vi "Read IMAQ Session.vi"(8 "error in (no error)":errorcluster, 10 "Camera Name":string, 11 "Gantry Class in":refnum<class "Gantry.lvclass">) -> (0 "error out":errorcluster, 2 "IMAQ Session":T1, 3 "Gantry Class out":refnum<class "Gantry.lvclass">)   [LabVIEW 2017, in "Gantry.lvclass"]
uses:
  Gantry.lvclass
  <vilib>/userdefined/High Color/IMAQdx.ctl
  Gantry.lvclass/Gantry.ctl
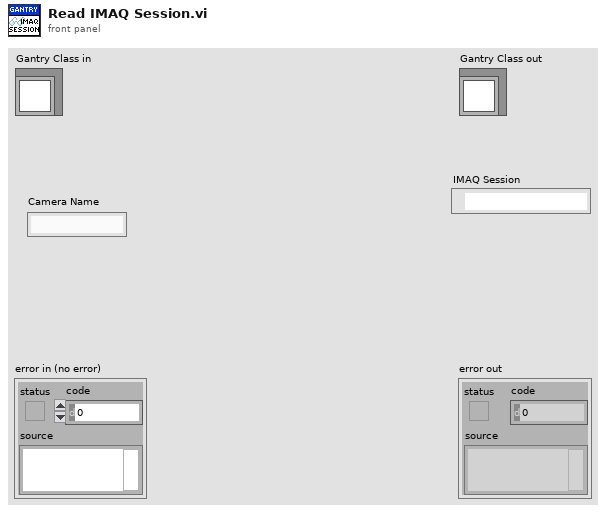
[diagram p1: front panel]
types:
  T1 = typedef "IMAQdx.ctl" = refnum<k21>
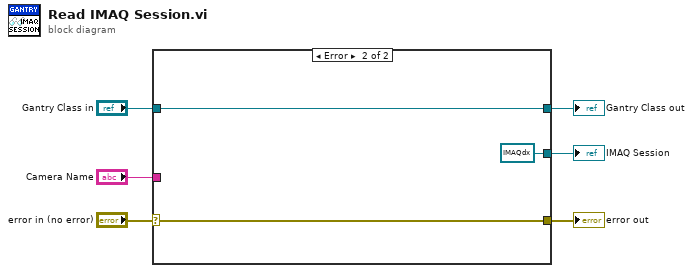
[diagram p0: block diagram]
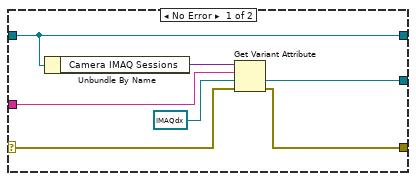
[diagram p2: hidden frame]
diagram:
  n1 = case shown="Error" "error in (no error)" {
    selector: "error in (no error)" -> [w10 w16]
    tunnel: [w8 w16] -> w5
    tunnel: [w13 w15] -> w3
    tunnel: "Gantry Class in" -> [w13 w15]
    tunnel: "Camera Name" -> [w11 _]
    tunnel: [w9 T1 refnum ("IMAQ Session")] -> w1
    frame No Error {
      n2 = Unbundle By Name(w13) -> ("Camera IMAQ Sessions"=w12:variant)
      n3 = Get Variant Attribute(Variant=w12, name=w11, default value (empty Variant)=T1 refnum ("IMAQ Session"), error in=w10) -> (value=w9:T1, error out=w8:errorcluster)  [unwired: 2 out]
    }
    frame Error {
    }
  }
  "error out" <- w5
  "Gantry Class out" <- w3
  "IMAQ Session" <- w1
